vi "Get Temperature.vi"(6 "Channel":i32, 8 "error in (no error)":errorcluster, 11 "instrument.PPMS":refnum<class "instrument.PPMS.lvclass">) -> (0 "error out":errorcluster, 1 "Status":string, 2 "Temperature (K)":dbl, 3 "instrument.PPMS out":refnum<class "instrument.PPMS.lvclass">, 4 "Finished?":bool)   [LabVIEW 2019, in "instrument.PPMS.lvclass"]
uses:
  instrument.PPMS.lvclass
  872d5e6e-7615-42de-8a57-f7e225904edc.vi/0ed01db7-3f86-41c9-b465-393c799b49b3.vi
  872d5e6e-7615-42de-8a57-f7e225904edc.vi/e75a5b47-9b5b-4ed0-a8e2-19f6ead7cafd.vi
  872d5e6e-7615-42de-8a57-f7e225904edc.vi/e75a5b47-9b5b-4ed0-a8e2-19f6ead7cafd.vi/03922cee-18a6-4d76-acb6-b19aaf8af5c8.vi
  872d5e6e-7615-42de-8a57-f7e225904edc.vi/e75a5b47-9b5b-4ed0-a8e2-19f6ead7cafd.vi/3953e4c8-1e7a-4e6f-a985-45aa81a6a810.vi
  <userlib>/LevyLab/Levylab Instruments/SMOs/RemoteControl/API/Remote Client.vi
  <vilib>/JDP Science/JSONtext/JSON text to Variant.vi
  <vilib>/JDP Science/JSONtext/LVClass Serializer/JSONtext LVClass Serializer.lvclass
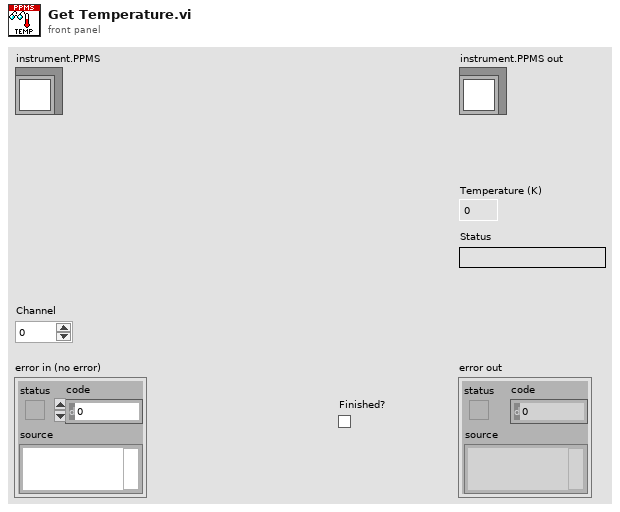
[diagram p1: front panel]
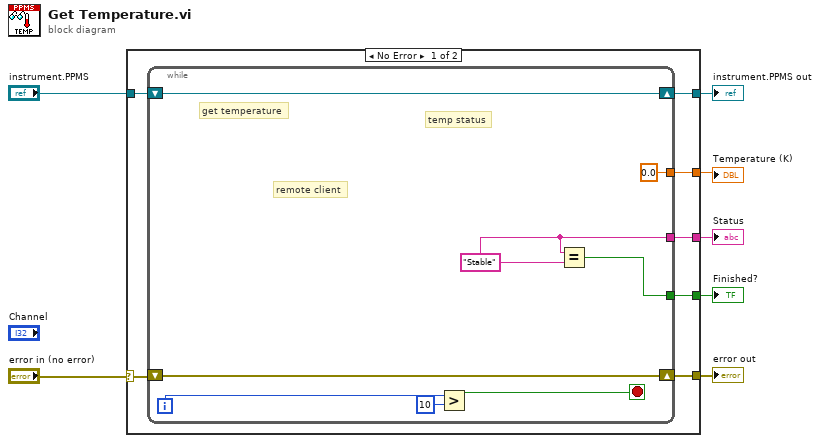
[diagram p0: block diagram]
diagram:
  n1 = case shown="No Error" "error in (no error)" {
    selector: "error in (no error)" -> [w8 w24]
    tunnel: [w14 _] -> w7
    tunnel: [w13 w24] -> w6
    tunnel: [w12 w23] -> w5
    tunnel: "instrument.PPMS" -> [w11 w23]
    tunnel: [w10 _] -> w3
    tunnel: [w9 _] -> w1
    frame No Error {
      n2 = while {
        tunnel: [0.0 ("Temperature (K)")] -> w14
        tunnel: [w17] -> w10
        shift-right: [w18] -> w13
        shift-left: w8 -> [w18]
        shift-right: [w19] -> w12
        shift-left: w11 -> [w19]
        tunnel: [w22] -> w9
        i -> [w20]
        stop <- w15 stop-if-true
        w17 = "Stable" ("Temperature Status")
        # "temp status"
        # "remote client"
        # "get temperature"
        n3 = Greater?(x=w20, y=10) -> (0:w15:bool)
        n4 = Equal?(x=w17, y=w17) -> (x = y?=w22:bool)
      }
    }
    frame Error {
    }
  }
  "error out" <- w6
  "instrument.PPMS out" <- w5
  "Temperature (K)" <- w7
  "Status" <- w3
  "Finished?" <- w1
